vi "Left Visible.vi"(8 "Current column":i32, 9 "Current row":i32, 10 "Full array":i32[][](array[numeric]), 11 "Element":i32) -> (2 "Viewing Distance":i32, 3 "Visible":bool)   [LabVIEW 2021]
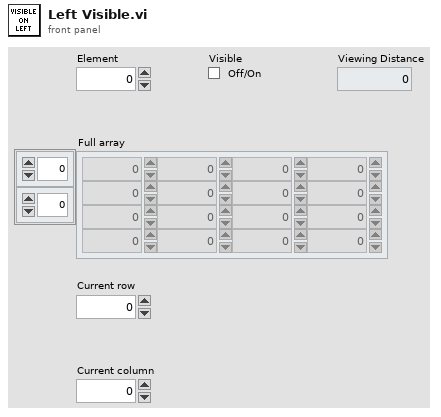
[diagram p1: front panel]
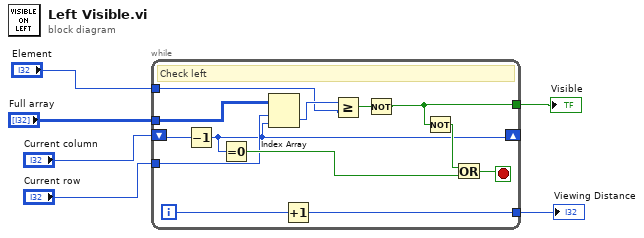
[diagram p0: block diagram]
diagram:
  n1 = while {
    shift-right: [w13] -> _
    shift-left: "Current column" -> [w19]
    tunnel: "Element" -> [w10]
    tunnel: "Full array" -> [w18]
    tunnel: "Current row" -> [w14]
    tunnel: [w9] -> w6
    tunnel: [w7] -> w1
    i -> [w8]
    stop <- w15 stop-if-true
    # "Check left"
    n2 = Decrement(x=w19) -> (x-1=w13:i32)
    n3 = Equal To 0?(x=w13) -> (x = 0?=w16:bool)
    n4 = Index Array(array=w18, index (row)=w14, index (col)=w13) -> (element=w11:i32)
    n5 = Increment(x=w8) -> (x+1=w7:i32)
    n6 = Greater Or Equal?(x=w11, y=w10) -> (x >= y?=w12:bool)
    n7 = Not(x=w12) -> (.not. x?=w9:bool)
    n8 = Not(x=w9) -> (.not. x?=w17:bool)
    n9 = Or(x=w17, y=w16) -> (x .or. y?=w15:bool)
  }
  "Visible" <- w6
  "Viewing Distance" <- w1
